vi "testclient.vi"() -> ()   [LabVIEW 2016]
uses:
  <vilib>/httpClient/LabVIEWHTTPClient.lvlib
panel:
  in  "Array":string[](array[string])=["http://username:password@localhost:80/path/data?key=value&key2=value2#fragid1", "http://localhost/absolute/URI/with/absolute/path/to/resource.txt", "http://localhost/scheme-relative/URI/with/absolute/path/to/resource.txt", "http://a:b@localhost/path/wah@t/foo.js?foo=bar&bingobang=&king=kong@kong.com#foobar/bing/bo@ng?bang"]
  out "x-y":dbl
  out "error out":errorcluster
  in  "Numeric 2":i32=1000
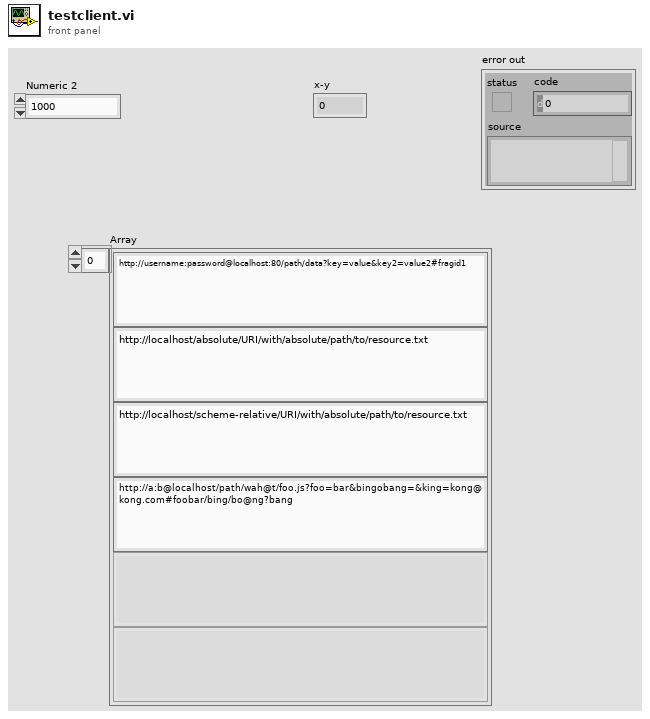
[diagram p1: front panel]
types:
  T1 = typedef "LabVIEWHTTPClient.lvlib/ClientHandle.ctl" = refnum<k1>
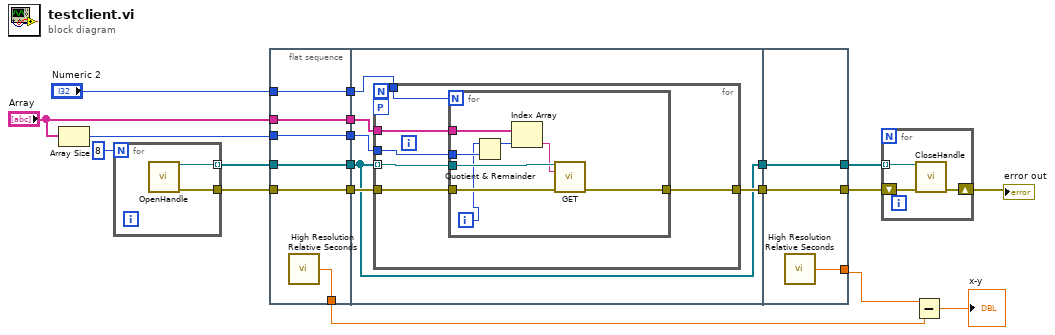
[diagram p0: block diagram]
diagram:
  n1 = Array Size(array="Array") -> (size(s)=w13:i32)
  n2 = for {
    N: 8 -> [_]
    tunnel: [w21] -> w19 mode=indexing
    tunnel: [w20] -> w17
    n3 = call <vilib>:"OpenHandle.vi"() -> ("client handle out"=w21:T1, "error out"=w20:errorcluster)  [unwired: 14 in]
  }
  n4 = flat-sequence {
    tunnel: "Array" -> [w23]
    tunnel: w13 -> [w24]
    tunnel: "Numeric 2" -> [w25]
    tunnel: w17 -> [w26]
    tunnel: w19 -> [w27]
    tunnel: [w27] -> w10
    tunnel: [w26] -> w9
    tunnel: [w25] -> w8
    tunnel: [w24] -> w7
    tunnel: [w23] -> w6
    tunnel: [w22] -> w4
    tunnel: [w32] -> w11
    tunnel: w10 -> [w29]
    tunnel: w9 -> [w33]
    tunnel: w8 -> [w28]
    tunnel: w7 -> [w31]
    tunnel: w6 -> [w30]
    tunnel: [w29] -> w3
    tunnel: [w49] -> w16
    tunnel: [w50] -> w18
    tunnel: w11 -> [w49]
    tunnel: [w48] -> w5
    tunnel: w3 -> [w50]
    frame #0 {
      n5 = call <vilib>:"High Resolution Relative Seconds.vi"() -> ("relative seconds"=w22:dbl)
    }
    frame #1 {
      n6 = for {
        tunnel: w31 -> [w36]
        tunnel: w30 -> [w35]
        workers-P: _ -> [_]
        tunnel: w29 -> [w39] mode=indexing
        tunnel: w33 -> [w38]
        tunnel: [w37] -> w32
        tunnel: w28 -> [w34]
        n7 = for {
          N: w34 -> [_]
          tunnel: w39 -> [w47]
          tunnel: w38 -> [w46]
          tunnel: [w45] -> w37
          tunnel: w36 -> [w44]
          tunnel: w35 -> [w42]
          i -> [w40]
          n8 = Quotient & Remainder(x=w40, y=w44) -> (x-y*floor(x/y)=w43:i32)  [unwired: 1 out]
          n9 = Index Array(array=w42, index=w43) -> (element=w41:string)
          n10 = call <vilib>:"GET.vi"("client handle"=w47, "url"=w41, "error in (no error)"=w46) -> ("error out"=w45:errorcluster)  [unwired: 9 in, 3 out]
        }
      }
    }
    frame #2 {
      n11 = call <vilib>:"High Resolution Relative Seconds.vi"() -> ("relative seconds"=w48:dbl)
    }
  }
  n12 = for {
    tunnel: w18 -> [w53] mode=indexing
    shift-right: [w51] -> w2
    shift-left: w16 -> [w52]
    n13 = call <vilib>:"CloseHandle.vi"("client handle"=w53, "error in (no error)"=w52) -> ("error out"=w51:errorcluster)  [unwired: 13 in]
  }
  "error out" <- w2
  n14 = Subtract(x=w5, y=w4) -> (x-y=→"x-y":dbl)
